vi "NI AO.vi"() -> ()   [LabVIEW 2019]
uses:
  <vilib>/Utility/error.llb/DialogType.ctl
  <instrlib>/Yokogawa DL950 Series/Yokogawa DL950 Series.lvlib
  cde7f783-3b1d-405b-9646-ac2e51606e9e.vi
  <instrlib>/Yokogawa DL950 Series/Public/Data/Read Waveform (Multiple).vi
  <vilib>/DAQmx/configure/timing.llb/DAQmx Timing (Sample Clock).vi
  <vilib>/DAQmx/write.llb/DAQmx Write (Analog 1D Wfm NChan NSamp).vi
  <vilib>/DAQmx/create/channels.llb/DAQmx Create Channel (AO-Voltage-Basic).vi
  <instrlib>/Yokogawa DL950 Series/Public/Configure/Configure Module (4-CH Voltage).vi
panel:
  out "R_max":dbl
  out "Response[s] 2":dbl
  out "Response[s] 1":dbl
  in  "Response time 2":dbl
  in  "Response time 1":dbl
  out "LoopTime(Total) 6":dbl=20.21659564971924
  out "LoopTime(Total) 5":dbl=20.26493215560913
  out "Ch 6":bool
  out "Ch 5":bool
  in  "samples per channel":i32=2000
  out "scope time(ms)":u32(slide)=2794 scale=0.0..5000.0
  out "size(s)":i32=10001
  out "ch":i32=2
  out "cycleControl":bool
  out "OffStart":bool=TRUE
  out "LoopTime(Total) 4":dbl=20.27935266494751
  out "LoopTime(Total) 3":dbl=20.197556972503662
  out "LoopTime(Total) 2":dbl=20.207571983337402
  out "LoopTime(Total)":dbl=20.261836528778076
  out "Cycle[N]":i32=156
  out "Discharge Relay":bool=TRUE
  out "Compute":bool
  out "DL950 Trigger":bool
  in  "Channel Enale(1: CH1)":u16[](array[ring])=[1, 1] items=["", "CH1", "CH2", "CH3", "CH4", "CH5", "CH6", "CH7", "CH8", "CH9", "CH10", "CH11", "CH12", "CH13", "CH14", "CH15", "CH16", "RMATH1", "RMATH2", "RMATH3", "RMATH4", "RMATH5", "RMATH6", "RMATH7", "RMATH8", "RMATH9", "RMATH10", "RMATH11", "RMATH12", "RMATH13", "RMATH14", "RMATH15", "RMATH16"]
  in  "Vertical Division (20: 50V)":i32(ring)=12 items=["0.1m", "0.2m", "0.5m", "1m", "2m", "5m", "10m", "20m", "50m", "100m", "200m", "500m", "1", "2", "4", "5", "8", "10", "20", "40", "50", "80", "100", "200", "400", "500", "800", "1k", "2k", "4k", "5k", "8k", "10k", "20k", "25k", "50k", "100k", "250k", "500k", "1000k"]
  in  "Probe Attenuation (3: 10:1)":i32(ring)=3 caption="Probe (10: 1)" items=["1:1", "2:1", "5:1", "10:1", "20:1", "50:1", "100:1", "200:1", "500:1", "1000:1", "2000:1", "5000:1", "10k:1", "20k:1", "50k:1", "0.1A:1V", "0.2A:1V", "0.5A:1V", "1A:1V", "2A:1V", "5A:1V", "10A:1V", "20A:1V", "50A:1V", "100A:1V", "200A:1V", "250A:1V", "400A:1V", "500A:1V", "1kA:1V", "2kA:1V", "5kA:1V", "10kA:1V", "20kA:1V", "50kA:1V", "NoSet"]
  in  "Vertical Coupling (1: DC)":i32(ring)=1 items=["AC", "DC", "Ground", "AC-RMS", "DC-RMS"]
  in  "Trigger Level (0)":dbl=0.5 format="%.3p"
  in  "Trigger Slope (0: Rising)":i32(ring) items=["Rising", "Falling", "Both"]
  in  "Trigger Mode (1: Auto)":i32(ring) items=["Normal", "Auto", "Auto Level", "Single", "Single(N)", "On Start", "No Set"]
  in  "Time Division (12: 1ms)":i32(ring)=19 items=["100ns", "200ns", "500ns", "1us", "2us", "5us", "10us", "20us", "50us", "100us", "200us", "500us", "1ms", "2ms", "5ms", "10ms", "20ms", "50ms", "100ms", "200ms", "500ms", "1s", "2s", "3s", "4s", "5s", "6s", "10s", "20s", "30s", "1min", "2min", "3min", "4min", "5min", "6min", "10min", "12min", "30min", "1hour", "2hour", "3hour", "4hour", "5hour", "6hour", "8hour", "10hour", "12hour", "1day", "2day", "3day", "4day", "5day"]
  in  "Acquisition Mode (0: Normal)":i32(ring) items=["Normal", "Average", "Envelope"]
  in  "Record Length (0: 10k)":i32(ring) items=["10k", "25k", "50k", "100k", "250k", "500k", "1M", "2.5M", "5M", "10M", "25M", "50M", "100M", "250M", "500M", "1G", "2G", "4G", "5G", "10G", "20G", "50G"]
  in  "trig source":i32[](array[ring])=[1, 1] items=["", "CH1", "CH2", "CH3", "CH4", "CH5", "CH6", "CH7", "CH8", "CH9", "CH10", "CH11", "CH12", "CH13", "CH14", "CH15", "CH16", "RMATH1", "RMATH2", "RMATH3", "RMATH4", "RMATH5", "RMATH6", "RMATH7", "RMATH8", "RMATH9", "RMATH10", "RMATH11", "RMATH12", "RMATH13", "RMATH14", "RMATH15", "RMATH16"]
  in  "channel":i32[](array[ring])=[1, 2] items=["", "CH1_1", "CH1_2", "CH2_1", "CH2_2", "CH3_1", "CH3_2", "CH4_1", "CH4_2", "CH5_1", "CH5_2", "CH6_1", "CH6_2", "CH7_1", "CH7_2", "CH8_1", "CH8_2", "CH9_1", "CH9_2", "CH10_1", "CH10_2", "CH11_1", "CH11_2", "CH12_1", "CH12_2", "CH13_1", "CH13_2", "CH14_1", "CH14_2", "CH15_1", "CH15_2", "CH16_1", "CH16_2"]
  in  "sub channel":u16[](array[ring])=[1, 2] items=["None", "SCH1", "SCH2", "SCH3", "SCH4", "SCH5", "SCH6", "SCH7", "SCH8", "SCH9", "SCH10", "SCH11", "SCH12", "SCH13", "SCH14", "SCH15", "SCH16", "SCH17", "SCH18", "SCH19", "SCH20", "SCH21", "SCH22", "SCH23", "SCH24", "SCH25", "SCH26", "SCH27", "SCH28", "SCH29", "SCH30", "SCH31", "SCH32", "SCH33", "SCH34", "SCH35", "SCH36", "SCH37", "SCH38", "SCH39", "SCH40", "SCH41", "SCH42", "SCH43", "SCH44", "SCH45", "SCH46", "SCH47", "SCH48", "SCH49", "SCH50", "SCH51", "SCH52", "SCH53", "SCH54", "SCH55", "SCH56", "SCH57", "SCH58", "SCH59", "SCH60", "SCH61", "SCH62", "SCH63", "SCH64"]
  in  "Hysteresis (1: Middle)":i32(ring) items=["Low", "Middle", "High"]
  in  "Source (1: CH1) 2":u16[](array[ring])=[1, 1] caption="Source (1: CH1)" items=["None", "CH1", "CH2", "CH3", "CH4", "CH5", "CH6", "CH7", "CH8", "CH9", "CH10", "CH11", "CH12", "CH13", "CH14", "CH15", "CH16", "MATH1", "MATH2", "MATH3", "MATH4", "MATH5", "MATH6", "MATH7", "MATH8", "EVENT"]
  in  "Sub Channel (0: None) 2":u16[](array[ring])=[1, 2] caption="Sub Channel (0: None)" items=["None", "SCH1", "SCH2", "SCH3", "SCH4", "SCH5", "SCH6", "SCH7", "SCH8", "SCH9", "SCH10", "SCH11", "SCH12", "SCH13", "SCH14", "SCH15", "SCH16", "SCH17", "SCH18", "SCH19", "SCH20", "SCH21", "SCH22", "SCH23", "SCH24", "SCH25", "SCH26", "SCH27", "SCH28", "SCH29", "SCH30", "SCH31", "SCH32", "SCH33", "SCH34", "SCH35", "SCH36", "SCH37", "SCH38", "SCH39", "SCH40", "SCH41", "SCH42", "SCH43", "SCH44", "SCH45", "SCH46", "SCH47", "SCH48", "SCH49", "SCH50", "SCH51", "SCH52", "SCH53", "SCH54", "SCH55", "SCH56", "SCH57", "SCH58", "SCH59", "SCH60", "SCH61", "SCH62", "SCH63", "SCH64"]
  in  "Enable Calibration (F: No)":bool
  in  "Enable Auto Setup (T: Yes)":bool
  in  "VISA resource name":refnum<visa-resource-name>="TCPIP0::192.168.0.100::inst0::INSTR"
  out "x-y":u32=3320
  in  "stop":bool
  out "Waveform Graph 2":waveform(dbl)[](graph)=[{"t0"=timestamp(0 s since 1904-01-01), "dt"=0.0002, "Y"=array[10001 elements]}, {"t0"=timestamp(0 s since 1904-01-01), "dt"=0.0002, "Y"=array[10001 elements]}]
  out "Power Relay":bool
  out "Power":bool=TRUE
  out "Ch 1":bool
  out "Ch 2":bool
  out "Ch 3":bool=TRUE
  out "Ch 4":bool
  out "loop time":u32=9
  out "Elapsed Time":dbl=0.9797806739807129
  in  "Sample Rate":dbl=2000.0
  in  "Sample Clock Source":tag="OnboardClock"
  out "Waveform Graph":waveform(dbl)[](graph)=[{"t0"=timestamp(0 s since 1904-01-01), "dt"=0.0005, "Y"=array[2000 elements]}, {"t0"=timestamp(0 s since 1904-01-01), "dt"=0.0005, "Y"=array[2000 elements]}]
  in  "Time(S)":dbl=0.8
  in  "c":dbl=0.001
  in  "r":dbl=4.0
  in  "v":dbl=4.0
  in  "Off Time":dbl=20.0
  in  "Stop":bool
  in  "Max Voltage":dbl=10.0
  in  "Min Voltage":dbl=-10.0
  in  "Physical Channel(s)":tag="cDAQ1Mod1/ao0:1"
  # "사이클 시간은 전채널 통일하고, \n전 채널 스캔방식으로 시험 제안"
  # "1. 방전릴레이 OFF: 100ms \n2. 파워릴레이 ON: 100ms\n3. 출력릴레이 ON: 100ms\n4. 스코프 트리거 대기\n5. 파워 ON\n6. 파워릴레이 OFF\n7. 파워 OFF\n8. 스코프 파형 수집 & 파형연산: 3000ms\n9. 출력릴레이 OFF: 100ms\n10. 방전릴레이 ON: 100ms\n11. 방전: 1000ms\n\n토탈 시간: 4500ms"
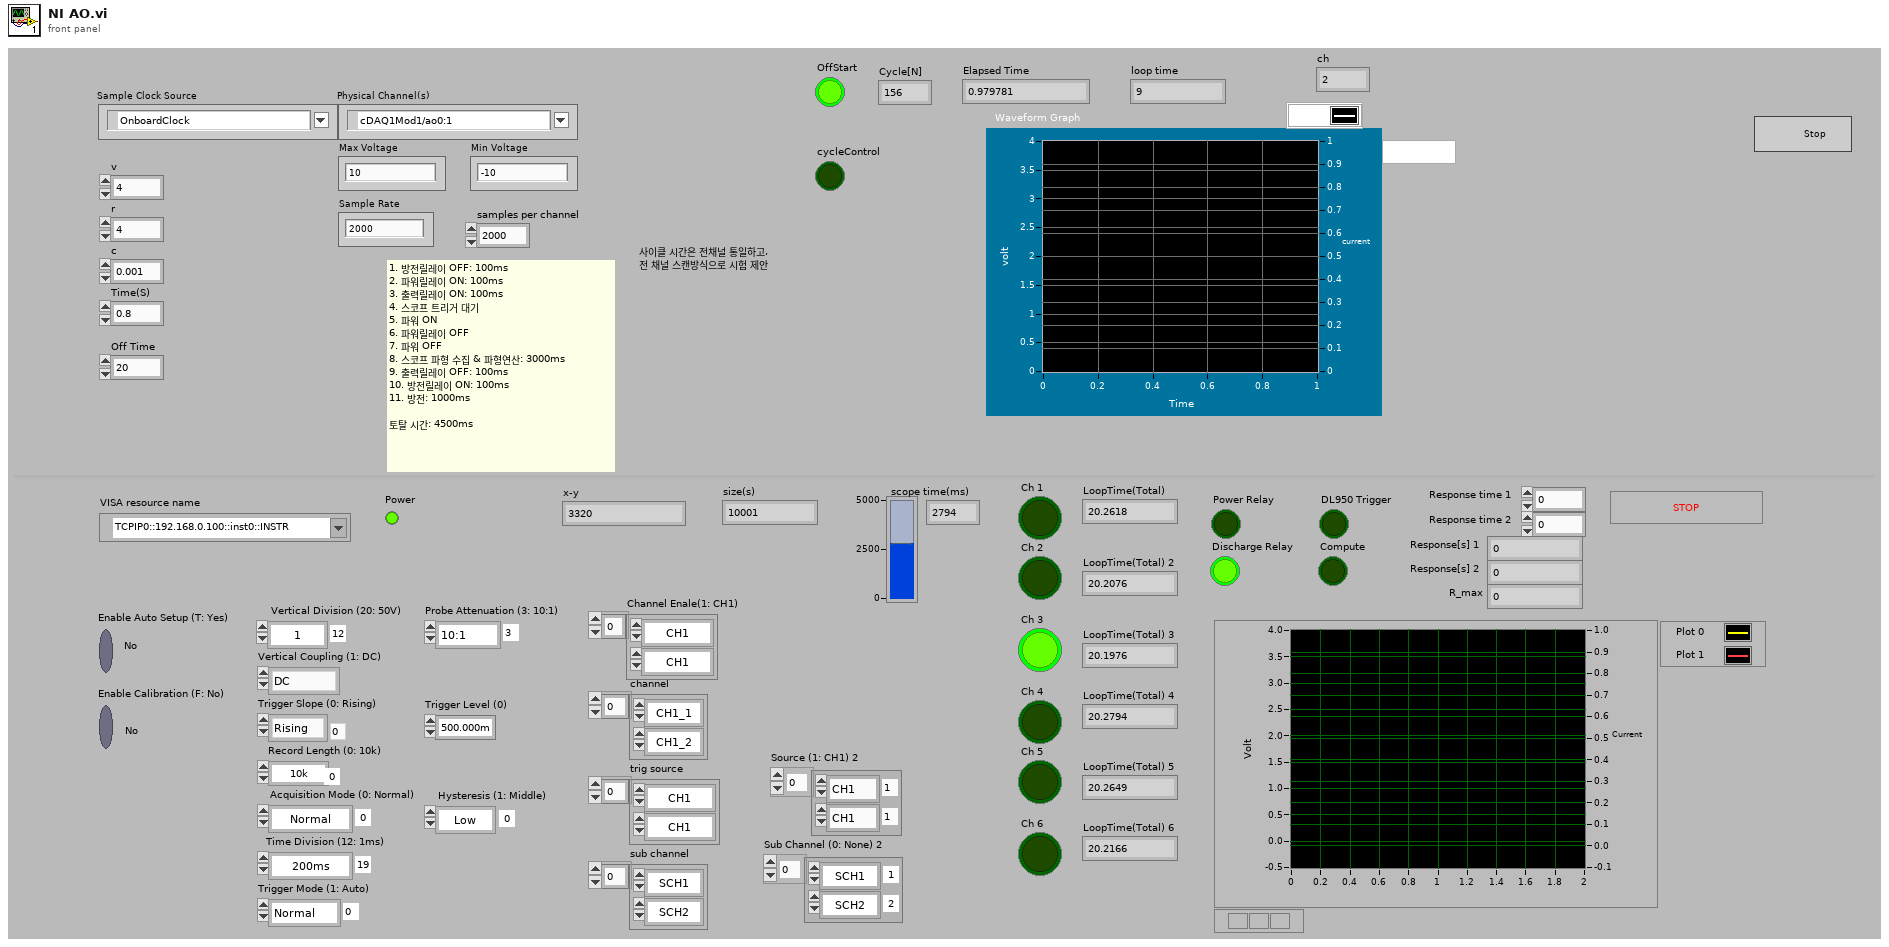
[diagram p1: front panel]
types:
  T1 = typedef "DialogType.ctl" = u16
  T2 = cluster{"pulse":i32, "Rising[%] 1":dbl, "Rising[%] 2":dbl, "Falling[%]":dbl, "R_max":dbl}
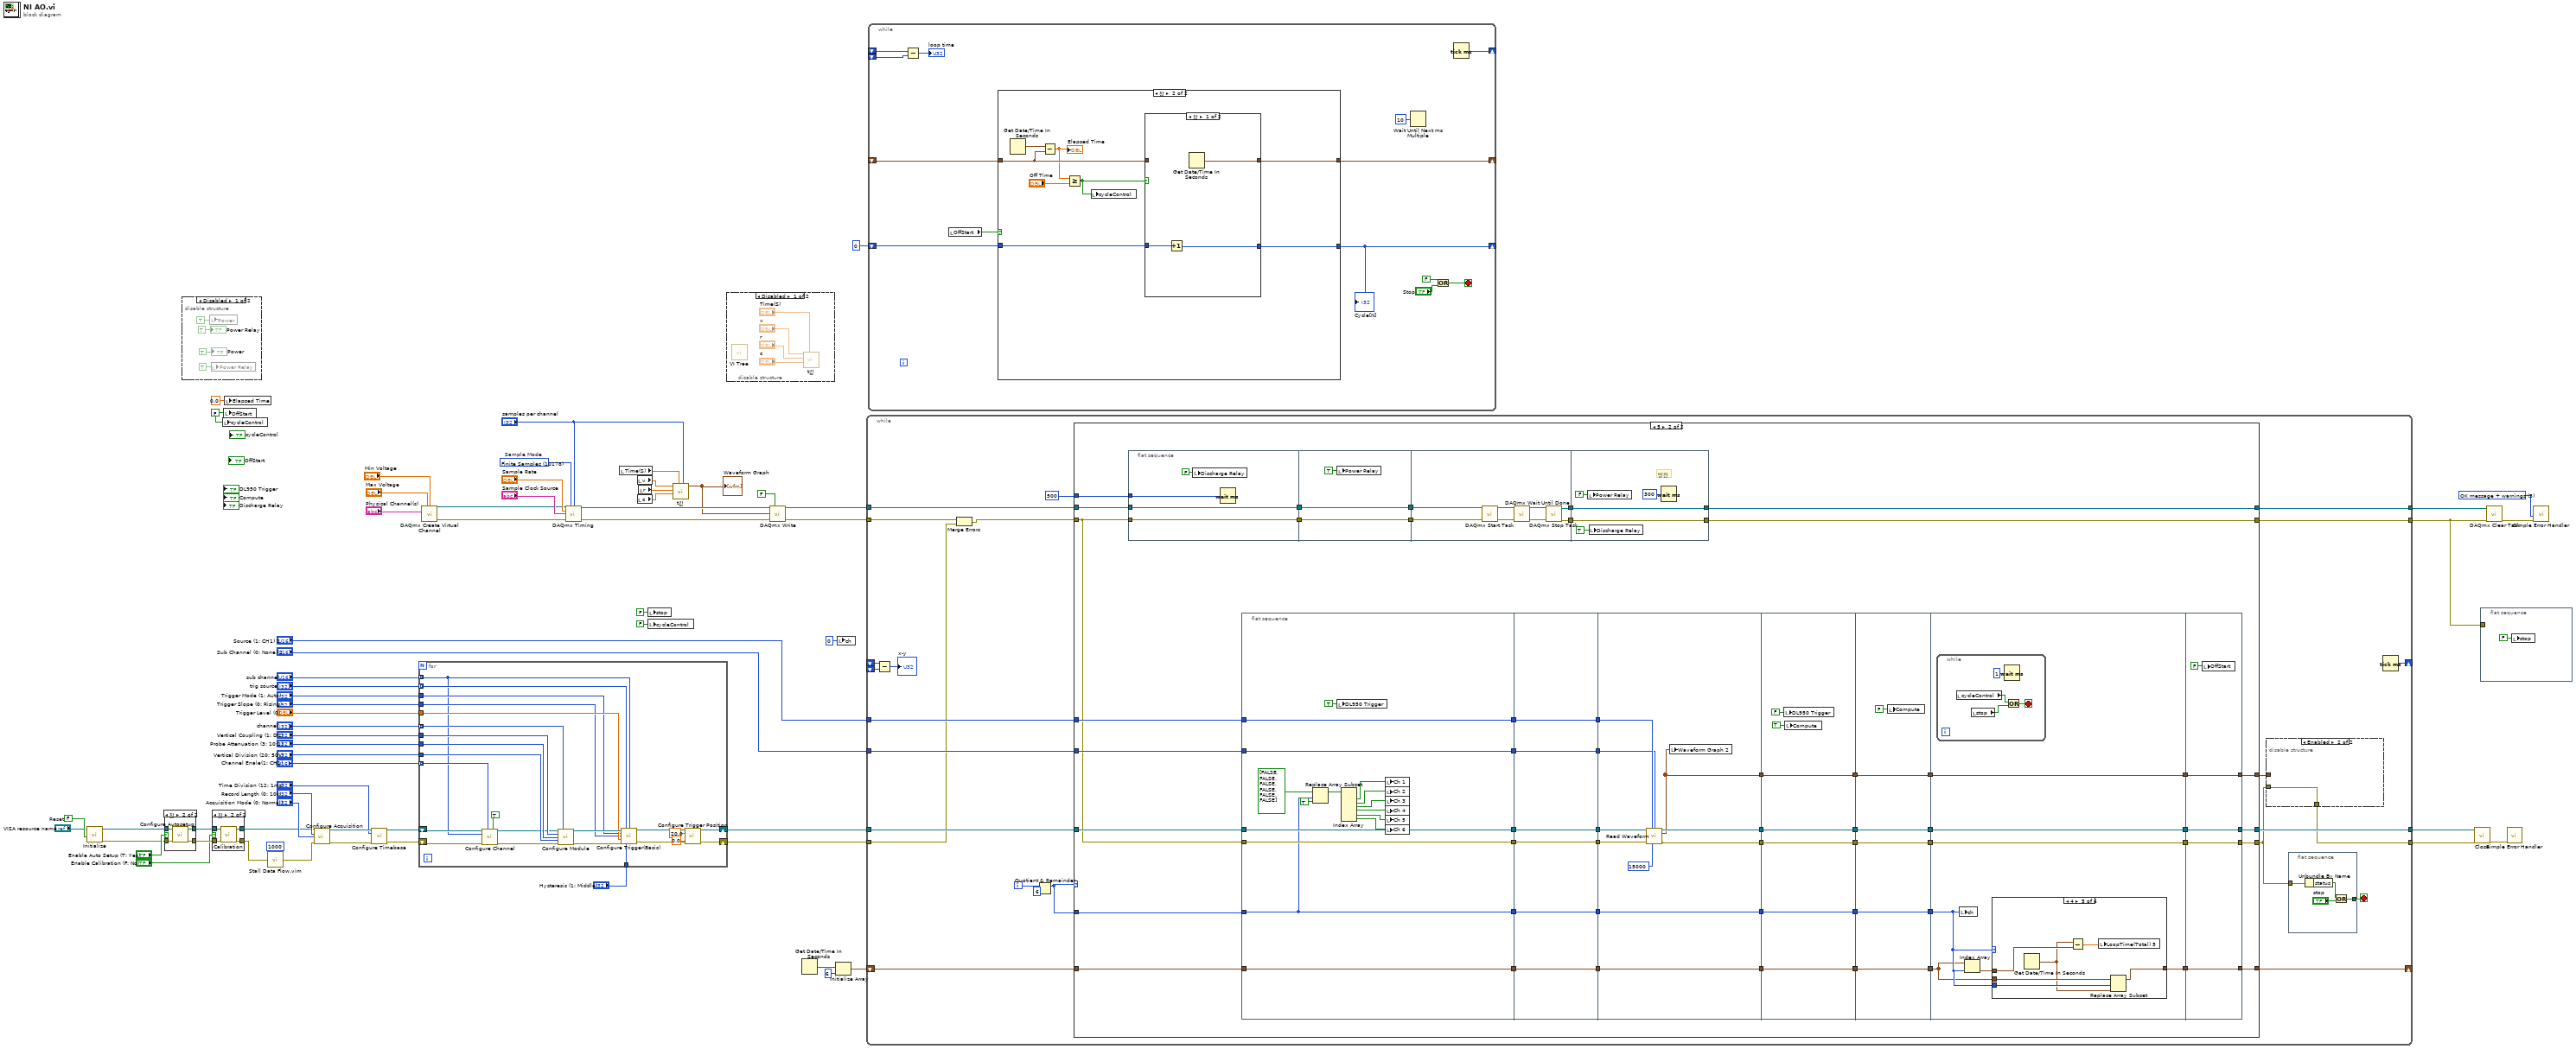
[diagram p0: block diagram]
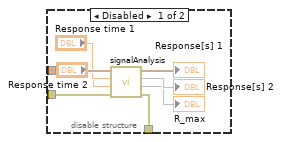
[diagram p6: hidden frame]
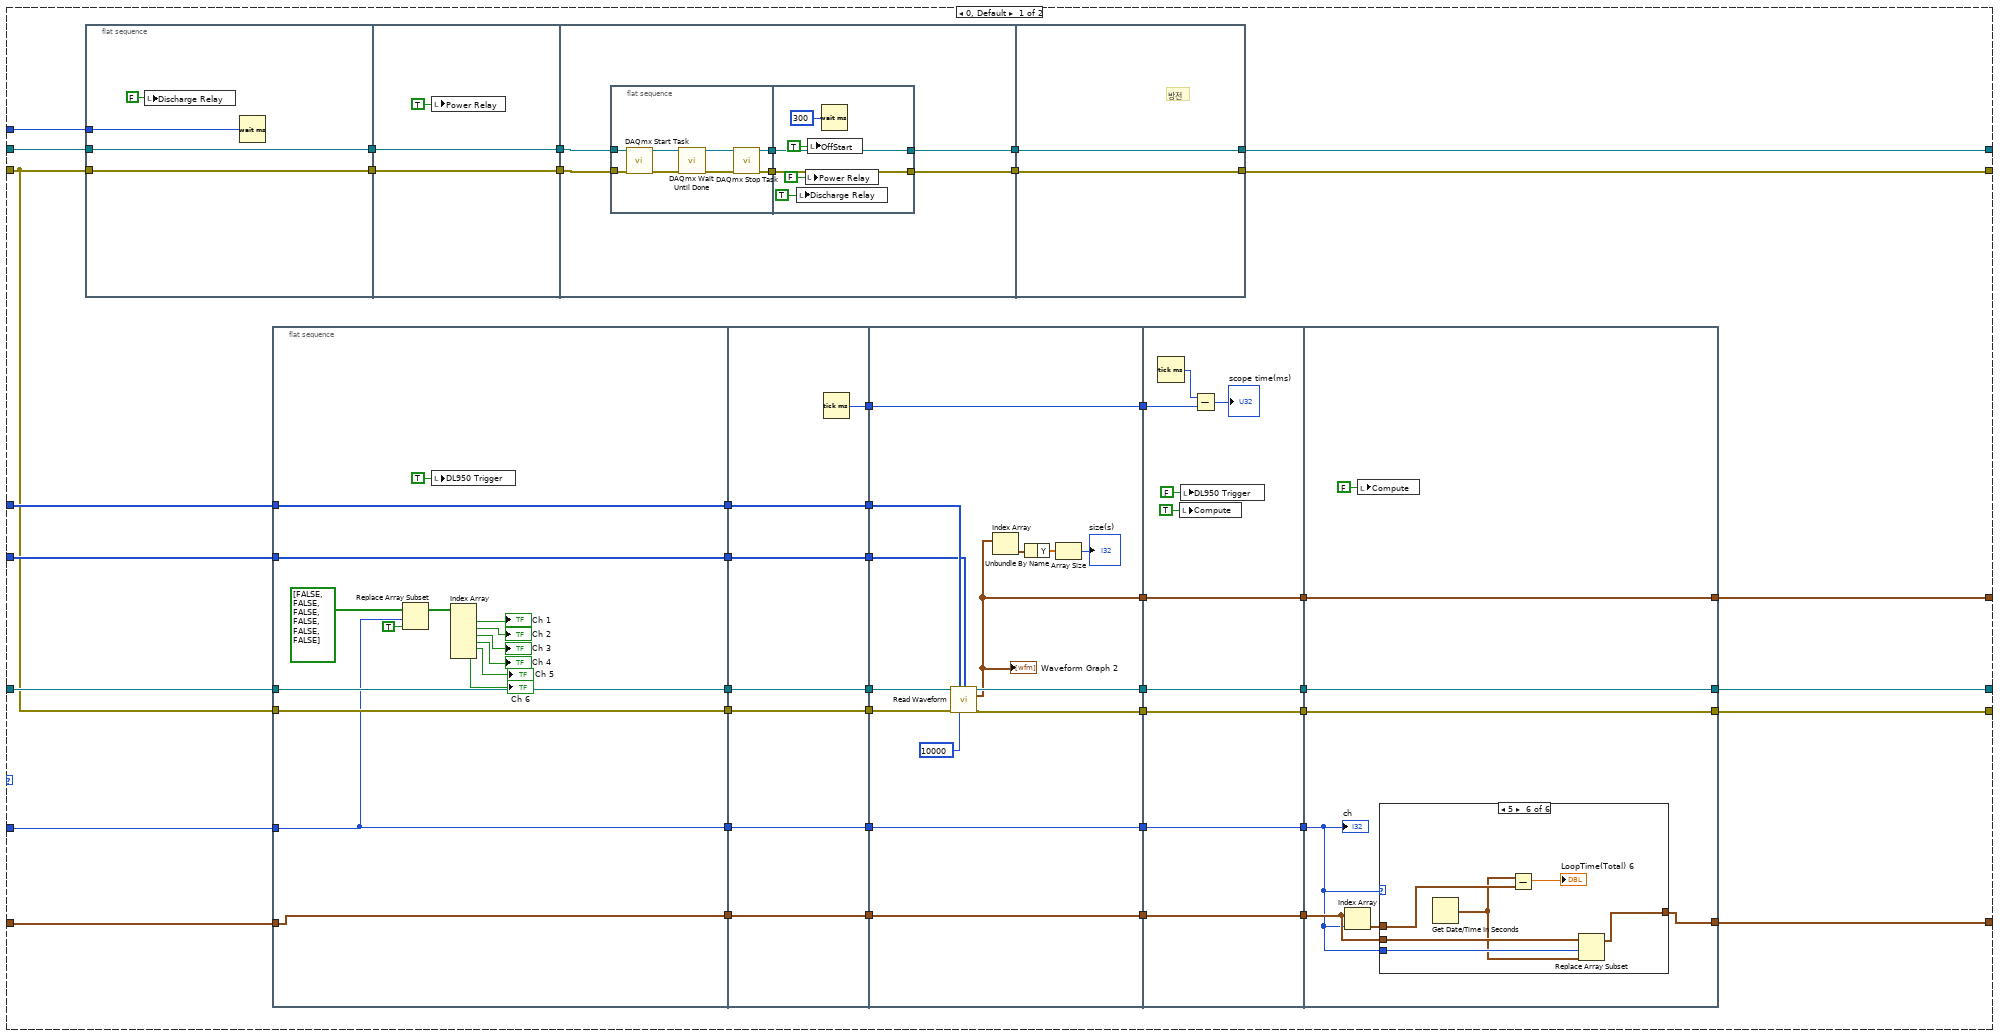
[diagram p7: hidden frame]
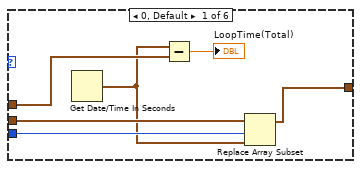
[diagram p8: hidden frame]
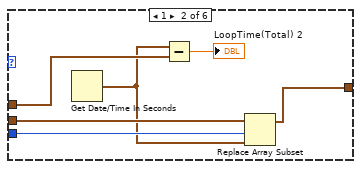
[diagram p9: hidden frame]
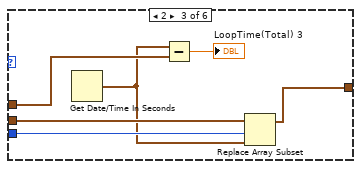
[diagram p10: hidden frame]
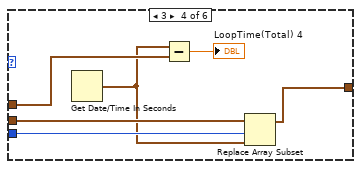
[diagram p11: hidden frame]
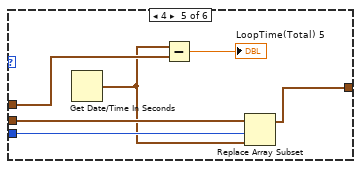
[diagram p12: hidden frame]
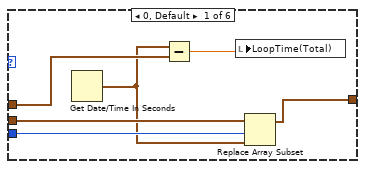
[diagram p13: hidden frame]
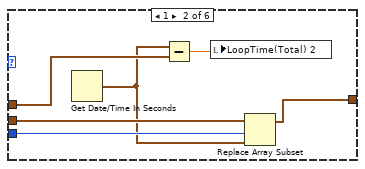
[diagram p14: hidden frame]
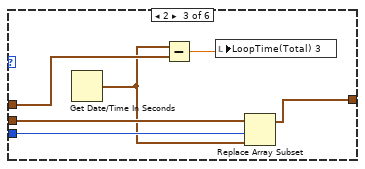
[diagram p15: hidden frame]
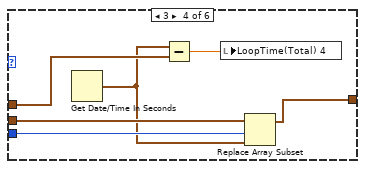
[diagram p16: hidden frame]
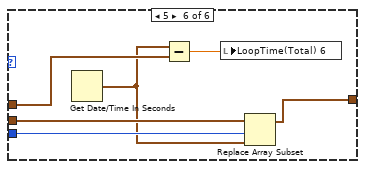
[diagram p17: hidden frame]
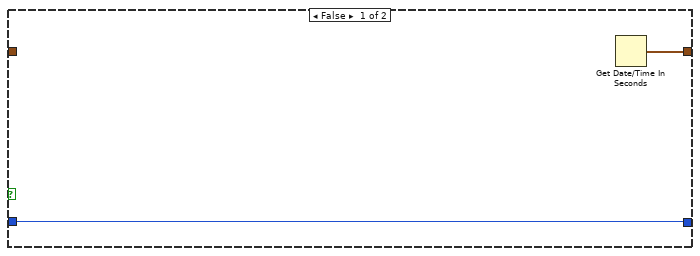
[diagram p18: hidden frame]
diagram:
  w6 = FALSE ("OffStart")
  w52 = FALSE  # Reset
  w59 = 10178 items=["Finite Samples"=10178, "Continuous Samples"=10123, "Hardware Timed Single Point"=12522]  # Sample Mode
  w65 = T1 3 items=["no dialog", "OK message", "continue or stop message", "OK message + warnings", "continue/stop + warnings"] ("type of dialog (OK msg:1)")
  n1 = call <instrlib>:"Initialize.vi"("Reset (True)"=w52, "VISA resource name"="VISA resource name") -> ("error out"=w19:errorcluster, "VISA resource name out"=w20:refnum<visa-resource-name>)  [unwired: 8 in]
  n2 = case shown="참" "Enable Auto Setup (T: Yes)" {
    tunnel: w20 -> [w71 w75]
    tunnel: [w71 w74] -> w48
    tunnel: w19 -> [w70 w73]
    tunnel: [w70 w72] -> w47
    frame False {
    }
    frame True {
      n3 = call <instrlib>:"Configure Autosetup.vi"("VISA resource name"=w75, "error in (no error)"=w73) -> ("VISA resource name out"=w74:refnum<visa-resource-name>, "error out"=w72:errorcluster)  [unwired: 12 in]
    }
  }
  n4 = disable-structure shown="Disabled" {
    frame Disabled {
      n5 = local write "Power"(TRUE ("Power")) -> ()
      n6 = local write "Power Relay"(TRUE ("Power Relay")) -> ()
      "Power" <- TRUE ("Power")
      "Power Relay" <- TRUE ("Power Relay")
    }
    frame Enabled {
    }
  }
  n7 = case shown="참" "Enable Calibration (F: No)" {
    tunnel: w48 -> [w81 w85]
    tunnel: [w81 w84] -> w18
    tunnel: w47 -> [w80 w83]
    tunnel: [w80 w82] -> w17
    frame False {
    }
    frame True {
      n8 = call <instrlib>:"Calibration.vi"("error in (no error)"=w83, "VISA resource name"=w85) -> ("error out"=w82:errorcluster, "VISA resource name out"=w84:refnum<visa-resource-name>)  [unwired: 8 in]
    }
  }
  n9 = local write "cycleControl"(w6) -> ()
  n10 = local write "OffStart"(w6) -> ()
  n11 = local write "Elapsed Time"(0.0 ("Elapsed Time")) -> ()
  n12 = call "Stall Data Flow.vim"("value in"=w17, "milliseconds to wait"=u32 1000) -> ("value out"=w16:errorcluster)  [unwired: 1 out]
  n13 = call <instrlib>:"Configure Acquisition.vi"("VISA resource name"=w18, "Record Length (0: 10k)"="Record Length (0: 10k)", "Acquisition Mode (0: Normal)"="Acquisition Mode (0: Normal)", "error in (no error)"=w16) -> ("VISA resource name out"=w39:refnum<visa-resource-name>, "error out"=w38:errorcluster)  [unwired: 10 in]
  n14 = call <instrlib>:"Configure Timebase.vi"("VISA resource name"=w39, "Time Division (12: 1ms)"="Time Division (12: 1ms)", "error in (no error)"=w38) -> ("VISA resource name out"=w37:refnum<visa-resource-name>, "error out"=w36:errorcluster)  [unwired: 11 in]
  n15 = for {
    tunnel: "channel" -> [w96] mode=indexing
    tunnel: "trig source" -> [w109] mode=indexing
    tunnel: "sub channel" -> [w92] mode=indexing
    tunnel: "Hysteresis (1: Middle)" -> [w108]
    shift-right: [w90] -> w22
    shift-left: w37 -> [w99]
    shift-right: [w88] -> w21
    shift-left: w36 -> [w97]
    tunnel: "Trigger Level (0)" -> [w105]
    tunnel: "Trigger Slope (0: Rising)" -> [w104]
    tunnel: "Trigger Mode (1: Auto)" -> [w103]
    tunnel: "Vertical Division (20: 50V)" -> [w102]
    tunnel: "Probe Attenuation (3: 10:1)" -> [w101]
    tunnel: "Vertical Coupling (1: DC)" -> [w100]
    tunnel: "Channel Enale(1: CH1)" -> [w94] mode=indexing
    n16 = call <instrlib>:"Configure Channel.vi"("VISA resource name"=w99, "Channel (1: CH1)"=w94, "Enable Channel (True)"=TRUE, 5:w92, "error in (no error)"=w97) -> ("VISA resource name out"=w98:refnum<visa-resource-name>, "error out"=w95:errorcluster)  [unwired: 9 in]
    n17 = call-poly <instrlib>:"Configure Module.vi"("VISA resource name"=w98, "Channel (1: CH1_1)"=w96, "Vertical Coupling (1: DC)"=w100, "Probe Attenuation (3: 10:1)"=w101, "Vertical Division (20: 50V)"=w102, "error in (no error)"=w95) -> ("VISA resource name out"=w107:refnum<visa-resource-name>, "error out"=w106:errorcluster)  [unwired: 8 in]
    n18 = call <instrlib>:"Configure Trigger(Basic).vi"("VISA resource name"=w107, "Trigger Source (1: CH1)"=w109, "Sub Channel (0: None)"=w92, "Trigger Mode (1: Auto)"=w103, "Trigger Slope (0: Rising)"=w104, "Trigger Level (0)"=w105, "error in (no error)"=w106, "Hysteresis (1: Middle)"=w108) -> ("VISA resource name out"=w91:refnum<visa-resource-name>, "error out"=w89:errorcluster)  [unwired: 6 in]
    n19 = call <instrlib>:"Configure Trigger Position.vi"("VISA resource name"=w91, "Trigger Position (50%)"=20.0, "Trigger Delay (0.0000000s)"=0.0, "error in (no error)"=w89) -> ("VISA resource name out"=w90:refnum<visa-resource-name>, "error out"=w88:errorcluster)  [unwired: 10 in]
  }
  n20 = call-poly <vilib>:"DAQmx Create Virtual Channel.vi"("maximum value"="Max Voltage", "minimum value"="Min Voltage", "physical channels"="Physical Channel(s)") -> ("task out"=w56:refnum<k21>, "error out"=w55:errorcluster)  [unwired: 11 in]
  n21 = call-poly <vilib>:"DAQmx Timing.vi"("task/channels in"=w56, "sample mode"=w59, "samples per channel"="samples per channel", "rate"="Sample Rate", "source"="Sample Clock Source", "error in"=w55) -> ("task out"=w54:refnum<k21>, "error out"=w53:errorcluster)  [unwired: 8 in]
  n22 = local read "Time(S)"() -> (w64:dbl)
  n23 = local read "v"() -> (w63:dbl)
  n24 = local read "c"() -> (w61:dbl)
  n25 = local read "r"() -> (w62:dbl)
  n26 = local write "stop"(FALSE ("stop")) -> ()
  n27 = local write "cycleControl"(FALSE ("cycleControl")) -> ()
  n28 = call "t값.vi"("samples"="samples per channel", "Time(S)"=w64, "c"=w61, "r"=w62, "v"=w63) -> ("Waveform Graph"=w13:waveform(dbl)[])  [unwired: 4 in, 2 out]
  "Waveform Graph" <- w13
  n29 = disable-structure shown="Disabled" {
    frame Disabled {
      n30 = call <instrlib>:"VI Tree.vi"() -> ()  [unwired: 12 in]
      n31 = call "t값.vi"("Time(S)"="Time(S)", "c"="c", "r"="r", "v"="v") -> ()  [unwired: 5 in, 3 out]
    }
    frame Enabled {
    }
  }
  n32 = call-poly <vilib>:"DAQmx Write.vi"("task/channels in"=w54, "auto start"=FALSE, "data"=w13, "error in"=w53) -> ("task out"=w15:refnum<k21>, "error out"=w14:errorcluster)  [unwired: 9 in, 1 out]
  n33 = Get Date/Time In Seconds() -> (seconds since 1Jan1904=w10:timestamp)
  n34 = Initialize Array(w10, 6 ("dimension size")) -> (w8:timestamp[])
  n35 = local write "ch"(0 ("ch")) -> ()
  n36 = while "Whileループ" {
    shift-right: [w137] -> _
    shift-left: _ -> [w136]
    shift-left: _ -> [w135]
    tunnel: w22 -> [w133]
    tunnel: w21 -> [w123]
    tunnel: "Source (1: CH1) 2" -> [w132]
    tunnel: "Sub Channel (0: None) 2" -> [w131]
    tunnel: [w130] -> w24
    tunnel: [w114] -> w23
    tunnel: w15 -> [w129]
    tunnel: w14 -> [w124]
    tunnel: [w128] -> w12
    tunnel: [w127] -> w2
    shift-right: [w126] -> _
    shift-left: w8 -> [w125]
    i -> [w119]
    stop <- w121 stop-if-true
    n37 = Subtract(x=w136, y=w135) -> (x-y=→"x-y":u32)
    n38 = Merge Errors(w124, w123) -> (w122:errorcluster)
    n39 = Quotient & Remainder(x=w119, y=6) -> (x-y*floor(x/y)=w118:i32)  [unwired: 1 out]
    n40 = case shown="5" w118 {
      tunnel: w133 -> [w176 w347]
      tunnel: w132 -> [w175 w346]
      tunnel: w131 -> [w174 w345]
      tunnel: [w173 w344] -> w130
      tunnel: [w172 w343] -> w115
      tunnel: w118 -> [w165 w342]
      tunnel: w129 -> [w171 w341]
      tunnel: [w170 w340] -> w128
      tunnel: [w169 w339] -> w127
      tunnel: [w168 w338] -> w126
      tunnel: w125 -> [w167 w337]
      tunnel: w122 -> [w166 w336]
      tunnel: u32 500 ("milliseconds to wait") -> [w162 w330]
      tunnel: [w161 w329] -> w116
      frame 0, Default {
        n41 = flat-sequence {
          tunnel: w166 -> [w197]
          tunnel: w171 -> [w198]
          tunnel: [w198] -> w182
          tunnel: [w197] -> w181
          tunnel: w162 -> [w195]
          tunnel: [w201] -> w180
          tunnel: [w199] -> w179
          tunnel: w182 -> [w201]
          tunnel: w181 -> [w199]
          tunnel: w180 -> [w207]
          tunnel: [w206] -> w178
          tunnel: w179 -> [w205]
          tunnel: [w204] -> w177
          tunnel: [w223] -> w170
          tunnel: w178 -> [w223]
          tunnel: [w222] -> w169
          tunnel: w177 -> [w222]
          frame #0 {
            n42 = local write "Discharge Relay"(FALSE ("Discharge")) -> ()
            n43 = Wait (ms)(milliseconds to wait=w195) -> ()  [unwired: 1 out]
          }
          frame #1 {
            n44 = local write "Power Relay"(TRUE ("Power Relay")) -> ()
          }
          frame #2 {
            n45 = flat-sequence {
              tunnel: w207 -> [w211]
              tunnel: w205 -> [w209]
              tunnel: [w210] -> w203
              tunnel: [w208] -> w202
              tunnel: [w220] -> w204
              tunnel: [w221] -> w206
              tunnel: w203 -> [w221]
              tunnel: w202 -> [w220]
              frame #0 {
                n46 = call <vilib>:"DAQmx Start Task.vi"("task/channels in"=w211, "error in"=w209) -> ("task out"=w213:refnum<k21>, "error out"=w212:errorcluster)  [unwired: 12 in]
                n47 = call <vilib>:"DAQmx Wait Until Done.vi"("task/channels in"=w213, "error in"=w212) -> ("task out"=w215:refnum<k21>, "error out"=w214:errorcluster)  [unwired: 12 in]
                n48 = call <vilib>:"DAQmx Stop Task.vi"("task/channels in"=w215, "error in"=w214) -> ("task out"=w210:refnum<k21>, "error out"=w208:errorcluster)  [unwired: 12 in]
              }
              frame #1 {
                n49 = local write "Discharge Relay"(TRUE ("Discharge")) -> ()
                n50 = local write "Power Relay"(FALSE ("Power Relay")) -> ()
                n51 = local write "OffStart"(TRUE ("OffStart")) -> ()
                n52 = Wait (ms)(milliseconds to wait=u32 300) -> ()  [unwired: 1 out]
              }
            }
          }
          frame #3 {
            # "방전"
          }
        }
        n53 = flat-sequence {
          tunnel: w176 -> [w239]
          tunnel: w166 -> [w238]
          tunnel: w175 -> [w237]
          tunnel: w174 -> [w236]
          tunnel: [w239] -> w194
          tunnel: [w238] -> w193
          tunnel: [w237] -> w192
          tunnel: [w236] -> w191
          tunnel: w167 -> [w224]
          tunnel: w165 -> [w225]
          tunnel: [w225] -> w155
          tunnel: [w224] -> w151
          tunnel: w194 -> [w246]
          tunnel: [w246] -> w190
          tunnel: w193 -> [w245]
          tunnel: [w245] -> w189
          tunnel: w192 -> [w244]
          tunnel: [w244] -> w188
          tunnel: w191 -> [w243]
          tunnel: [w243] -> w187
          tunnel: [w242] -> w163
          tunnel: [w241] -> w156
          tunnel: w155 -> [w241]
          tunnel: [w240] -> w152
          tunnel: w151 -> [w240]
          tunnel: w190 -> [w257]
          tunnel: w189 -> [w256]
          tunnel: w188 -> [w259]
          tunnel: w187 -> [w258]
          tunnel: [w255] -> w186
          tunnel: [w254] -> w185
          tunnel: [w250] -> w164
          tunnel: w163 -> [w250]
          tunnel: [w249] -> w159
          tunnel: [w248] -> w157
          tunnel: w156 -> [w248]
          tunnel: [w247] -> w153
          tunnel: w152 -> [w247]
          tunnel: w186 -> [w270]
          tunnel: w185 -> [w269]
          tunnel: [w270] -> w184
          tunnel: [w269] -> w183
          tunnel: w164 -> [w265]
          tunnel: [w263] -> w160
          tunnel: w159 -> [w263]
          tunnel: [w262] -> w158
          tunnel: w157 -> [w262]
          tunnel: [w261] -> w154
          tunnel: w153 -> [w261]
          tunnel: w184 -> [w278]
          tunnel: w183 -> [w276]
          tunnel: [w278] -> w173
          tunnel: [w276] -> w172
          tunnel: [w272] -> w168
          tunnel: [w275] -> w161
          tunnel: w160 -> [w275]
          tunnel: w158 -> [w271]
          tunnel: w154 -> [w273]
          frame #0 {
            n54 = Replace Array Subset(array=bool[] [FALSE, FALSE, FALSE, FALSE, FALSE, FALSE], new element=TRUE ("new element/subarray"), index=w225) -> (w235:bool[])
            n55 = local write "DL950 Trigger"(TRUE ("DL950 Trigger")) -> ()
            n56 = Index Array(array=w235) -> (element #1=→"Ch 1":bool, element #2=→"Ch 2":bool, element #3=→"Ch 3":bool, element #4=→"Ch 4":bool, element #5=→"Ch 5":bool, element #6=→"Ch 6":bool)  [unwired: 6 in]
          }
          frame #1 {
            n57 = Tick Count (ms)() -> (millisecond timer value=w242:u32)
          }
          frame #2 {
            n58 = call-poly <instrlib>:"Read Waveform.vi"("VISA resource name"=w257, "Source (1: CH1)"=w259, "Sub Channel (0: None)"=w258, "error in (no error)"=w256, "Timeout (10000 ms)"=u32 10000) -> ("VISA resource name out"=w255:refnum<visa-resource-name>, "Waveform Data"=w249:waveform(dbl)[], "error out"=w254:errorcluster)  [unwired: 8 in]
            "Waveform Graph 2" <- w249
            n59 = Index Array(array=w249) -> (element=w253:waveform(dbl))  [unwired: 1 in]
            n60 = Unbundle By Name(w253) -> ("Y"=w252:dbl[])
            n61 = Array Size(array=w252) -> (size(s)=→"size(s)":i32)
          }
          frame #3 {
            n62 = Tick Count (ms)() -> (millisecond timer value=w266:u32)
            n63 = local write "Compute"(TRUE ("Compute")) -> ()
            n64 = local write "DL950 Trigger"(FALSE ("DL950 Trigger")) -> ()
            n65 = Subtract(x=w266, y=w265) -> (x-y=→"scope time(ms)":u32)
          }
          frame #4 {
            n66 = Index Array(array=w273, index=w271) -> (element=w274:timestamp)
            n67 = local write "Compute"(FALSE ("Compute")) -> ()
            n68 = case shown="5" w271 {
              tunnel: [w279 w285 w291 w297 w304 w310] -> w272
              tunnel: w274 -> [w284 w290 w296 w302 w308 w314]
              tunnel: w273 -> [w282 w288 w294 w300 w307 w313]
              tunnel: w271 -> [w281 w287 w293 w299 w306 w312]
              frame 0, Default {
                n69 = Get Date/Time In Seconds() -> (seconds since 1Jan1904=w280:timestamp)
                n70 = Subtract(x=w280, y=w284) -> (x-y=→"LoopTime(Total)":dbl)
                n71 = Replace Array Subset(array=w282, new element=w280, index=w281) -> (w279:timestamp[])
              }
              frame 1 {
                n72 = Get Date/Time In Seconds() -> (seconds since 1Jan1904=w286:timestamp)
                n73 = Subtract(x=w286, y=w290) -> (x-y=→"LoopTime(Total) 2":dbl)
                n74 = Replace Array Subset(array=w288, new element=w286, index=w287) -> (w285:timestamp[])
              }
              frame 2 {
                n75 = Get Date/Time In Seconds() -> (seconds since 1Jan1904=w292:timestamp)
                n76 = Subtract(x=w292, y=w296) -> (x-y=→"LoopTime(Total) 3":dbl)
                n77 = Replace Array Subset(array=w294, new element=w292, index=w293) -> (w291:timestamp[])
              }
              frame 3 {
                n78 = Get Date/Time In Seconds() -> (seconds since 1Jan1904=w298:timestamp)
                n79 = Subtract(x=w298, y=w302) -> (x-y=→"LoopTime(Total) 4":dbl)
                n80 = Replace Array Subset(array=w300, new element=w298, index=w299) -> (w297:timestamp[])
              }
              frame 4 {
                n81 = Get Date/Time In Seconds() -> (seconds since 1Jan1904=w305:timestamp)
                n82 = Subtract(x=w305, y=w308) -> (x-y=→"LoopTime(Total) 5":dbl)
                n83 = Replace Array Subset(array=w307, new element=w305, index=w306) -> (w304:timestamp[])
              }
              frame 5 {
                n84 = Get Date/Time In Seconds() -> (seconds since 1Jan1904=w311:timestamp)
                n85 = Subtract(x=w311, y=w314) -> (x-y=→"LoopTime(Total) 6":dbl)
                n86 = Replace Array Subset(array=w313, new element=w311, index=w312) -> (w310:timestamp[])
              }
            }
            "ch" <- w271
          }
        }
      }
      frame 5 {
        n87 = flat-sequence {
          tunnel: w336 -> [w368]
          tunnel: w341 -> [w369]
          tunnel: [w369] -> w353
          tunnel: [w368] -> w352
          tunnel: w330 -> [w366]
          tunnel: [w372] -> w351
          tunnel: [w370] -> w350
          tunnel: w353 -> [w372]
          tunnel: w352 -> [w370]
          tunnel: w351 -> [w376]
          tunnel: [w375] -> w349
          tunnel: w350 -> [w374]
          tunnel: [w373] -> w348
          tunnel: [w385] -> w340
          tunnel: w349 -> [w385]
          tunnel: [w383] -> w339
          tunnel: w348 -> [w383]
          frame #0 {
            n88 = local write "Discharge Relay"(FALSE ("Discharge")) -> ()
            n89 = Wait (ms)(milliseconds to wait=w366) -> ()  [unwired: 1 out]
          }
          frame #1 {
            n90 = local write "Power Relay"(TRUE ("Power Relay")) -> ()
          }
          frame #2 {
            n91 = call <vilib>:"DAQmx Start Task.vi"("task/channels in"=w376, "error in"=w374) -> ("task out"=w378:refnum<k21>, "error out"=w377:errorcluster)  [unwired: 12 in]
            n92 = call <vilib>:"DAQmx Wait Until Done.vi"("task/channels in"=w378, "error in"=w377) -> ("task out"=w380:refnum<k21>, "error out"=w379:errorcluster)  [unwired: 12 in]
            n93 = call <vilib>:"DAQmx Stop Task.vi"("task/channels in"=w380, "error in"=w379) -> ("task out"=w375:refnum<k21>, "error out"=w373:errorcluster)  [unwired: 12 in]
          }
          frame #3 {
            # "방전"
            n94 = local write "Power Relay"(FALSE ("Power Relay")) -> ()
            n95 = local write "Discharge Relay"(TRUE ("Discharge")) -> ()
            n96 = Wait (ms)(milliseconds to wait=u32 300) -> ()  [unwired: 1 out]
          }
        }
        n97 = flat-sequence {
          tunnel: w347 -> [w401]
          tunnel: w336 -> [w400]
          tunnel: w346 -> [w399]
          tunnel: w345 -> [w398]
          tunnel: [w401] -> w365
          tunnel: [w400] -> w364
          tunnel: [w399] -> w363
          tunnel: [w398] -> w362
          tunnel: w342 -> [w387]
          tunnel: w337 -> [w386]
          tunnel: [w387] -> w320
          tunnel: [w386] -> w315
          tunnel: w365 -> [w407]
          tunnel: [w407] -> w361
          tunnel: w364 -> [w406]
          tunnel: [w406] -> w360
          tunnel: w363 -> [w405]
          tunnel: [w405] -> w359
          tunnel: w362 -> [w404]
          tunnel: [w404] -> w358
          tunnel: [w403] -> w321
          tunnel: w320 -> [w403]
          tunnel: [w402] -> w316
          tunnel: w315 -> [w402]
          tunnel: w361 -> [w414]
          tunnel: w360 -> [w413]
          tunnel: w359 -> [w416]
          tunnel: w358 -> [w415]
          tunnel: [w412] -> w357
          tunnel: [w411] -> w356
          tunnel: [w410] -> w325
          tunnel: [w409] -> w322
          tunnel: w321 -> [w409]
          tunnel: [w408] -> w317
          tunnel: w316 -> [w408]
          tunnel: w357 -> [w424]
          tunnel: w356 -> [w423]
          tunnel: [w424] -> w355
          tunnel: [w423] -> w354
          tunnel: [w420] -> w326
          tunnel: w325 -> [w420]
          tunnel: [w419] -> w323
          tunnel: w322 -> [w419]
          tunnel: [w418] -> w318
          tunnel: w317 -> [w418]
          tunnel: w355 -> [w430]
          tunnel: w354 -> [w428]
          tunnel: [w430] -> w335
          tunnel: [w428] -> w334
          tunnel: [w427] -> w327
          tunnel: w326 -> [w427]
          tunnel: [w426] -> w324
          tunnel: w323 -> [w426]
          tunnel: [w425] -> w319
          tunnel: w318 -> [w425]
          tunnel: w335 -> [w437]
          tunnel: w334 -> [w436]
          tunnel: [w437] -> w333
          tunnel: [w436] -> w332
          tunnel: [w431] -> w331
          tunnel: [w435] -> w328
          tunnel: w327 -> [w435]
          tunnel: w324 -> [w433]
          tunnel: w319 -> [w432]
          tunnel: [w480] -> w338
          tunnel: [w481] -> w343
          tunnel: [w482] -> w344
          tunnel: w333 -> [w482]
          tunnel: w332 -> [w481]
          tunnel: w331 -> [w480]
          tunnel: [w478] -> w329
          tunnel: w328 -> [w478]
          frame #0 {
            n98 = Replace Array Subset(array=bool[] [FALSE, FALSE, FALSE, FALSE, FALSE, FALSE], new element=TRUE ("new element/subarray"), index=w387) -> (w397:bool[])
            n99 = local write "DL950 Trigger"(TRUE ("DL950 Trigger")) -> ()
            n100 = Index Array(array=w397) -> (element #1=w393:bool, element #2=w392:bool, element #3=w391:bool, element #4=w390:bool, element #5=w389:bool, element #6=w388:bool)  [unwired: 6 in]
            n101 = local write "Ch 1"(w393) -> ()
            n102 = local write "Ch 2"(w392) -> ()
            n103 = local write "Ch 3"(w391) -> ()
            n104 = local write "Ch 4"(w390) -> ()
            n105 = local write "Ch 5"(w389) -> ()
            n106 = local write "Ch 6"(w388) -> ()
          }
          frame #1 {
          }
          frame #2 {
            n107 = call-poly <instrlib>:"Read Waveform.vi"("VISA resource name"=w414, "Source (1: CH1)"=w416, "Sub Channel (0: None)"=w415, "error in (no error)"=w413, "Timeout (10000 ms)"=u32 15000) -> ("VISA resource name out"=w412:refnum<visa-resource-name>, "Waveform Data"=w410:waveform(dbl)[], "error out"=w411:errorcluster)  [unwired: 8 in]
            n108 = local write "Waveform Graph 2"(w410) -> ()
          }
          frame #3 {
            n109 = local write "DL950 Trigger"(FALSE ("DL950 Trigger")) -> ()
            n110 = local write "Compute"(TRUE ("Compute")) -> ()
          }
          frame #4 {
            n111 = local write "Compute"(FALSE ("Compute")) -> ()
          }
          frame #5 {
            n112 = while {
              stop <- w474 stop-if-true
              n113 = local read "cycleControl"() -> (w476:bool)
              n114 = local read "stop"() -> (w475:bool)
              n115 = Wait (ms)(milliseconds to wait=u32 1) -> ()  [unwired: 1 out]
              n116 = Or(x=w476, y=w475) -> (x .or. y?=w474:bool)
            }
            n117 = local write "ch"(w433) -> ()
            n118 = Index Array(array=w432, index=w433) -> (element=w434:timestamp)
            n119 = case shown="4" w433 {
              tunnel: [w439 w445 w451 w457 w463 w469] -> w431
              tunnel: w434 -> [w443 w449 w455 w461 w467 w473]
              tunnel: w432 -> [w442 w448 w454 w460 w466 w472]
              tunnel: w433 -> [w441 w447 w453 w459 w465 w471]
              frame 0, Default {
                n120 = Get Date/Time In Seconds() -> (seconds since 1Jan1904=w440:timestamp)
                n121 = Subtract(x=w440, y=w443) -> (x-y=w438:dbl)
                n122 = local write "LoopTime(Total)"(w438) -> ()
                n123 = Replace Array Subset(array=w442, new element=w440, index=w441) -> (w439:timestamp[])
              }
              frame 1 {
                n124 = Get Date/Time In Seconds() -> (seconds since 1Jan1904=w446:timestamp)
                n125 = Subtract(x=w446, y=w449) -> (x-y=w444:dbl)
                n126 = local write "LoopTime(Total) 2"(w444) -> ()
                n127 = Replace Array Subset(array=w448, new element=w446, index=w447) -> (w445:timestamp[])
              }
              frame 2 {
                n128 = Get Date/Time In Seconds() -> (seconds since 1Jan1904=w452:timestamp)
                n129 = Subtract(x=w452, y=w455) -> (x-y=w450:dbl)
                n130 = local write "LoopTime(Total) 3"(w450) -> ()
                n131 = Replace Array Subset(array=w454, new element=w452, index=w453) -> (w451:timestamp[])
              }
              frame 3 {
                n132 = Get Date/Time In Seconds() -> (seconds since 1Jan1904=w458:timestamp)
                n133 = Subtract(x=w458, y=w461) -> (x-y=w456:dbl)
                n134 = local write "LoopTime(Total) 4"(w456) -> ()
                n135 = Replace Array Subset(array=w460, new element=w458, index=w459) -> (w457:timestamp[])
              }
              frame 4 {
                n136 = Get Date/Time In Seconds() -> (seconds since 1Jan1904=w464:timestamp)
                n137 = Subtract(x=w464, y=w467) -> (x-y=w462:dbl)
                n138 = local write "LoopTime(Total) 5"(w462) -> ()
                n139 = Replace Array Subset(array=w466, new element=w464, index=w465) -> (w463:timestamp[])
              }
              frame 5 {
                n140 = Get Date/Time In Seconds() -> (seconds since 1Jan1904=w470:timestamp)
                n141 = Subtract(x=w470, y=w473) -> (x-y=w468:dbl)
                n142 = local write "LoopTime(Total) 6"(w468) -> ()
                n143 = Replace Array Subset(array=w472, new element=w470, index=w471) -> (w469:timestamp[])
              }
            }
          }
          frame #6 {
            n144 = local write "OffStart"(FALSE ("OffStart")) -> ()
          }
        }
      }
    }
    n145 = disable-structure shown="Enabled" {
      disable-tunnel: w116 -> [w145 _]
      disable-tunnel: w115 -> [w144 w146]
      disable-tunnel: [w143 w146] -> w114
      frame Disabled {
        n146 = call "signalAnalysis.vi"("error in (no error)"=w144, "inpuPara"="Response time 2", "data_scope"="Response time 1", "출력 전압 전류 특성"=w145) -> ("error out"=w143:errorcluster, 1:→"R_max", 2:→"Response[s] 2", "data"=→"Response[s] 1":T2)  [unwired: 4 in]
      }
      frame Enabled {
      }
    }
    n147 = flat-sequence {
      tunnel: w115 -> [w148]
      tunnel: [w147] -> w121
      frame #0 {
        n148 = Unbundle By Name ("名前でバンドル解除")(w148) -> ("status"=w149:bool)
        n149 = Or(x=w149, y="stop") -> (x .or. y?=w147:bool)
      }
    }
    n150 = Tick Count (ms)() -> (millisecond timer value=w137:u32)
  }
  n151 = while {
    shift-right: [w494] -> _
    shift-left: _ -> [w493]
    shift-right: [w490] -> _
    shift-left: _ -> [w489]
    shift-left: _ -> [w488]
    shift-right: [w484] -> _
    shift-left: 0 -> [w485]
    stop <- w491 stop-if-true
    n152 = Subtract(x=w489, y=w488) -> (x-y=→"loop time":u32)
    n153 = local read "OffStart"() -> (w483:bool)
    n154 = case shown="참" w483 {
      tunnel: [w496 w505] -> w494
      tunnel: w493 -> [_ w504]
      tunnel: w485 -> [w497 w500]
      tunnel: [w497 w499] -> w484
      frame False {
        n155 = Get Date/Time In Seconds() -> (seconds since 1Jan1904=w496:timestamp)
      }
      frame True {
        n156 = Get Date/Time In Seconds() -> (seconds since 1Jan1904=w503:timestamp)
        n157 = Subtract(x=w503, y=w504) -> (x-y=w502:dbl)
        "Elapsed Time" <- w502
        n158 = Greater Or Equal?(x=w502, y="Off Time") -> (x >= y?=w498:bool)
        n159 = local write "cycleControl"(w498) -> ()
        n160 = case shown="참" w498 {
          tunnel: [w508 w510] -> w505
          tunnel: w504 -> [_ w510]
          tunnel: w500 -> [w507 w509]
          tunnel: [w506 w509] -> w499
          frame True {
            n161 = Increment(x=w507) -> (x+1=w506:i32)
            n162 = Get Date/Time In Seconds() -> (seconds since 1Jan1904=w508:timestamp)
          }
          frame False {
          }
        }
      }
    }
    "Cycle[N]" <- w484
    n163 = Wait Until Next ms Multiple(millisecond multiple=u32 10) -> ()  [unwired: 1 out]
    n164 = Or(x=FALSE, y="Stop") -> (x .or. y?=w491:bool)
    n165 = Tick Count (ms)() -> (millisecond timer value=w490:u32)
  }
  n166 = call <instrlib>:"Close.vi"("error in (no error)"=w23, "VISA resource name"=w24) -> ("error out"=w51:errorcluster)  [unwired: 9 in]
  n167 = flat-sequence {
    tunnel: w2 -> [_]
    frame #0 {
      n168 = local write "stop"(FALSE ("stop")) -> ()
    }
  }
  n169 = call <vilib>:"DAQmx Clear Task.vi"("task in"=w12, "error in"=w2) -> ("error out"=w69:errorcluster)  [unwired: 13 in]
  n170 = call <vilib>:"Simple Error Handler.vi"("error in (no error)"=w51) -> ()  [unwired: 4 in, 5 out]
  n171 = call <vilib>:"Simple Error Handler.vi"("type of dialog (OK msg:1)"=w65, "error in (no error)"=w69) -> ()  [unwired: 3 in, 5 out]
